vi "Stop Core.vi"(10 "final error code":i32, 11 "Measure Object in":refnum<class "Template Module.lvclass">) -> (3 "Measure Object out":refnum<class "Template Module.lvclass">)   [LabVIEW 2021, in "Template Module.lvclass"]
doc: "(<B>Filename</B>: Actor Framework.lvlib:Actor.lvclass:Stop Core.vi)\n\nDefines what the actor does before it stops. Use the <B>final error code</B> input to determine whether the actor shut down in response to an error.\n\nBy default, this method does nothing. A descendant class may override it to define behavior, such as shutting down any processes the actor initiated in its override of the Actor Core method."
uses:
  Template Module.lvclass
  Template Module.lvclass/Template Module.ctl
  <vilib>/ActorFramework/Actor/Actor.lvclass
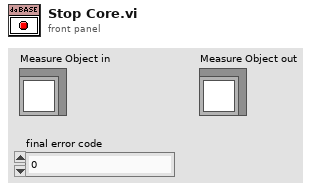
[diagram p1: front panel]
types:
  T1 = enum32{"Invalid", "Standard", "Closed", "Hidden", "Minimized", "Maximized"}
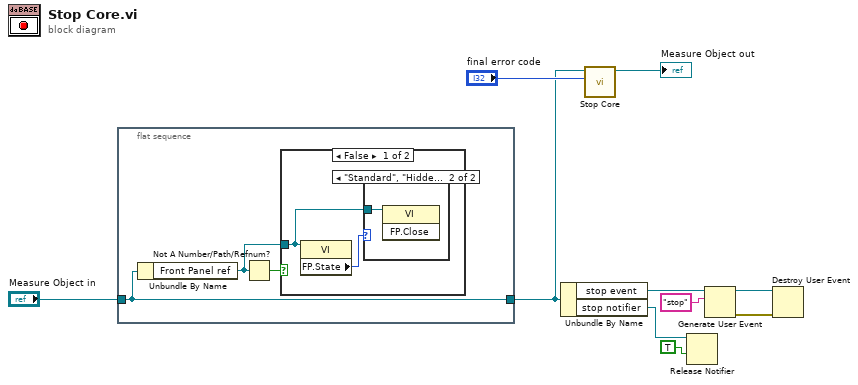
[diagram p0: block diagram]
diagram:
  n1 = flat-sequence {
    tunnel: "Measure Object in" -> [w13]
    tunnel: [w13] -> w1
    frame #0 {
      n2 = Unbundle By Name(w13) -> ("Front Panel ref"=w12:refnum<vi>)
      n3 = Not A Number/Path/Refnum?(number/path/refnum=w12) -> (NaN/Path/Refnum?=w11:bool)
      n4 = case shown="False" w11 {
        tunnel: w12 -> [w15 _]
        frame False {
          n5 = property class="VI"(reference=w15) -> ("FP.State"=w14:T1)  [unwired: 1 in, 2 out]
          n6 = case shown="\"Standard\", \"Hidden\"..\"Maximized\"" w14 {
            tunnel: w15 -> [_ w16]
            frame "Invalid", Default {
            }
            frame "Standard", "Hidden".."Maximized" {
              n7 = invoke class="VI" method="FP.Close"(reference=w16) -> ()  [unwired: 2 in, 3 out]
            }
          }
        }
        frame True {
        }
      }
    }
  }
  n8 = Unbundle By Name(w1) -> ("stop event"=w4:refnum<user-event>, "stop notifier"=w3:refnum<notifier>)
  n9 = call-parent "Stop Core.vi"("final error code"="final error code", "Actor in"=w1) -> ("Actor out"=→"Measure Object out":refnum<class "Template Module.lvclass">)  [unwired: 9 in]
  n10 = Release Notifier(notifier=w3, force destroy? (F)=TRUE) -> ()  [unwired: 1 in, 3 out]
  n11 = Generate User Event(user event=w4, event data cluster="stop" ("event data")) -> (user event out=w5:refnum<user-event>, error out=w6:errorcluster)  [unwired: 2 in]
  n12 = Destroy User Event(user event=w5, error in=w6) -> ()  [unwired: 1 out]
